vi "SA Reference Level Configuration - NF.vi"(8 "error in":errorcluster, 10 "RFmx Settings":T1={"RFmx Name"="", "RFmx Port"="", "Reference Level"={"DUT Max Gain (dB)"=0.0, "DUT Max Noise Figure (dB)"=0.0, "Mode"=enum."Manual", "Reference Level (dBm)"=0.0}, "Preamp Enabled"=0, "Attenuation"={"Mode"=enum."Constant Attenuation", "Constant Attenuation"={"RFmx External Attenuation (dB)"=11.2}, "s2p File"={"RFmx S-Parameters Orientation"=24000, "RFmx Attenuation s2p File"=path ""}}, "ENS Source"={"SMU Name"="", "SMU Channel"=""}} {"Attenuation"."s2p File"."RFmx S-Parameters Orientation" items=["Port1 Towards DUT"=24000, "Port2 Towards DUT"=24001]; "Attenuation"."Constant Attenuation"."RFmx External Attenuation (dB)" format="%.2f"; "Preamp Enabled" items=["Disabled"=0, "Enabled"=1, "Automatic"=3]}, 11 "RFmx Session in":refnum<k21>) -> (0 "error out":errorcluster, 3 "RFmx Session out":refnum<k21>)   [LabVIEW 2023]
uses:
  Controls/RFmx Config - NF.ctl
  <resource>/objmgr/RFmxSpecAn.rc
panel:
  out "Reference Level":dbl
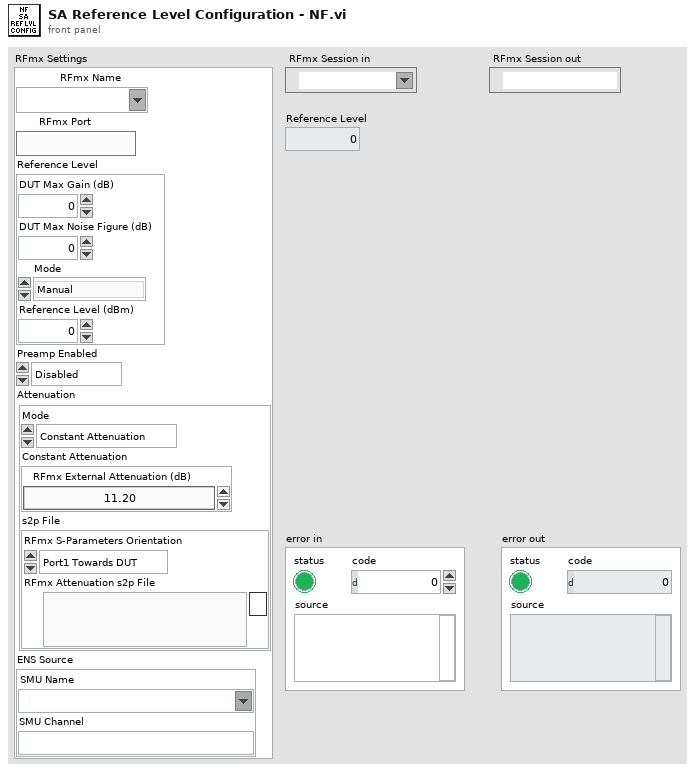
[diagram p1: front panel]
types:
  T1 = typedef "RFmx Config - NF.ctl" = cluster{"RFmx Name":refnum<k15>, "RFmx Port":string, "Reference Level":cluster{"DUT Max Gain (dB)":dbl, "DUT Max Noise Figure (dB)":dbl, "Mode":enum32{"Manual", "Recommend"}, "Reference Level (dBm)":dbl}, "Preamp Enabled":i32, "Attenuation":cluster{"Mode":enum32{"<None>", "Constant Attenuation", "s2p File"}, "Constant Attenuation":cluster{"RFmx External Attenuation (dB)":dbl}, "s2p File":cluster{"RFmx S-Parameters Orientation":i32, "RFmx Attenuation s2p File":path}}, "ENS Source":cluster{"SMU Name":refnum<k15>, "SMU Channel":string}}
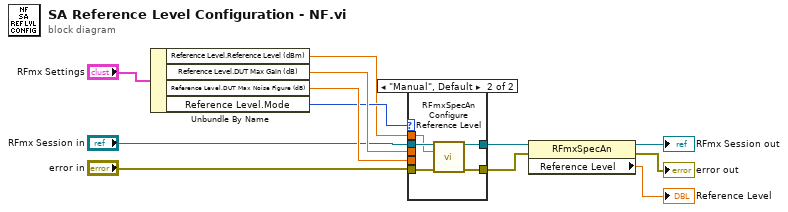
[diagram p0: block diagram]
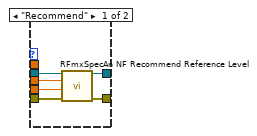
[diagram p2: hidden frame]
diagram:
  n1 = Unbundle By Name("RFmx Settings") -> ("Reference Level.Reference Level (dBm)"=w8:dbl, "Reference Level.DUT Max Gain (dB)"=w11:dbl, "Reference Level.DUT Max Noise Figure (dB)"=w12:dbl, "Reference Level.Mode"=w10:enum32{"Manual", "Recommend"})
  n2 = case shown="\"Manual\", Default" w10 {
    tunnel: "error in" -> [w18 w23]
    tunnel: [w17 w22] -> w2
    tunnel: "RFmx Session in" -> [w16 w20]
    tunnel: [w15 w21] -> w5
    tunnel: w8 -> [_ w19]
    tunnel: w11 -> [w14 _]
    tunnel: w12 -> [w13 _]
    frame "Recommend" {
      # "19.1"
      n3 = call <vilib>:"RFmxSpecAn NF Recommend Reference Level.vi"("Instrument Handle In"=w16, "DUT Max Gain (dB)"=w14, "DUT Max Noise Figure (dB)"=w13, "error in (no error)"=w18) -> ("Instrument Handle Out"=w15:refnum<k21>, "error out"=w17:errorcluster)  [unwired: 9 in, 1 out]
    }
    frame "Manual", Default {
      # "19.2"
      n4 = call <vilib>:"RFmxSpecAn Configure Reference Level.vi"("Instrument Handle In"=w20, "Reference Level"=w19, "error in (no error)"=w23) -> ("Instrument Handle Out"=w21:refnum<k21>, "error out"=w22:errorcluster)  [unwired: 11 in]
    }
  }
  n5 = property class="RFmxSpecAn"(reference=w5, error in=w2) -> (reference out=→"RFmx Session out":refnum<k21>, error out=→"error out":errorcluster, "Reference Level"=→"Reference Level":dbl)
